vi "Get best pixel array.vi"(9 "Cell details cluster":T1={"Measure?"=TRUE, "Area (cm^2)"=0.0, "Cell Label"="", "Cell Description"="", "Cell Position"=0, "Time in rig (s)"=16.0, "Time to next scan (s)"=0.0, "Scan number"=1.0, "When did you stick it in?"=0.0, "Time between scans (s)"=0.0, "Time of the last scan (s)"=0.0, "Scan settings in queue"=0, "Sample Holder"=0.0, "User Name"=""} {"Scan settings in queue" items=["Regular", "Inverted", "MartinaSettings"]; "Time of the last scan (s)" format="%<%H:%M:%S>t"; "When did you stick it in?" format="%<%H:%M:%S>t"; "Time to next scan (s)" format="%<%H:%M:%S>t"; "Time in rig (s)" format="%<%H:%M:%S>t"}, 10 "Number of best pixels":dbl, 11 "File path of master log":path) -> (2 "Pixel Array":dbl[](array[numeric]), 3 "Vmp Array":dbl[](array[numeric]))   [LabVIEW 2011]
uses:
  Typedefs/Queue cluster.ctl
  <vilib>/Utility/file.llb/Read From Spreadsheet File (string).vi
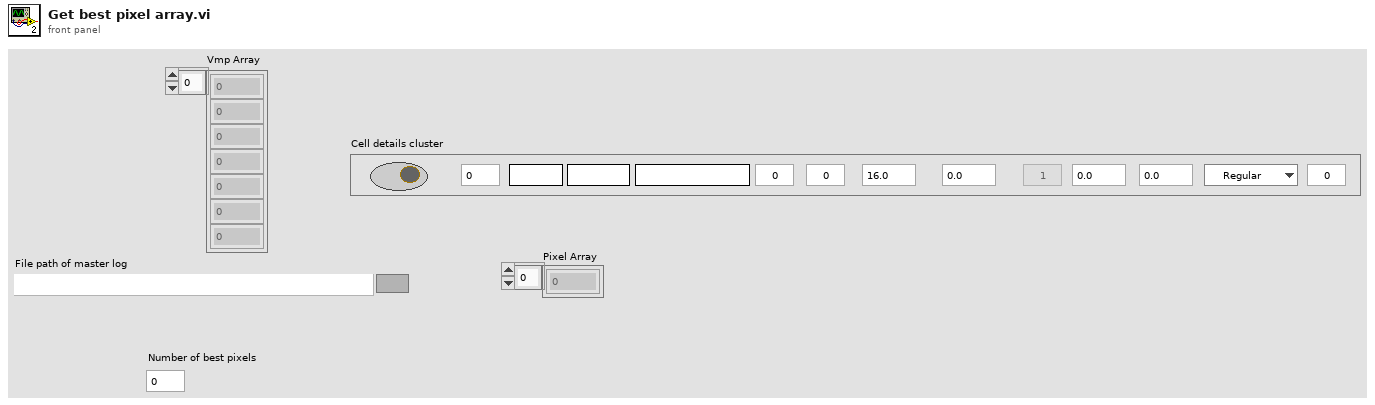
[diagram p1: front panel]
types:
  T1 = typedef "Queue cluster.ctl" = cluster{"Measure?":bool, "Area (cm^2)":dbl, "Cell Label":string, "Cell Description":string, "Cell Position":i32, "Time in rig (s)":dbl, "Time to next scan (s)":dbl, "Scan number":dbl, "When did you stick it in?":dbl, "Time between scans (s)":dbl, "Time of the last scan (s)":dbl, "Scan settings in queue":u16, "Sample Holder":dbl, "User Name":string}
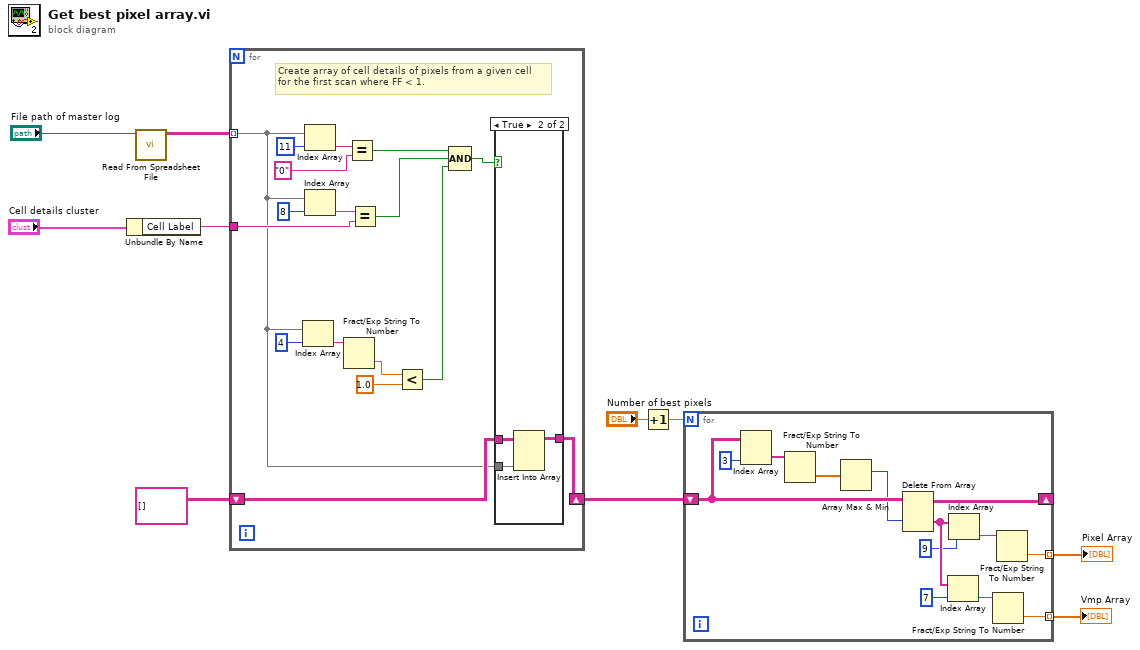
[diagram p0: block diagram]
diagram:
  n1 = Unbundle By Name("Cell details cluster") -> ("Cell Label"=w2:string)
  n2 = call-poly <vilib>:"Read From Spreadsheet File.vi"("file path (dialog if empty)"="File path of master log") -> ("all rows"=w9:string[][])  [unwired: 6 in, 4 out]
  n3 = for {
    tunnel: w9 -> [w12] mode=indexing
    shift-right: [w24] -> w7
    shift-left: string[][] [] ("all rows") -> [w25]
    tunnel: w2 -> [w20]
    # "Create array of cell details of pixels from a given cell\nfor the first scan where FF < 1."
    n4 = Index Array(array=w12, index=4) -> (element=w15:string)
    n5 = Index Array(array=w12, index=11) -> (element=w26:string)
    n6 = Index Array(array=w12, index=8) -> (element=w21:string)
    n7 = Fract/Exp String To Number(string=w15) -> (number=w14:dbl)  [unwired: 3 in, 1 out]
    n8 = Equal?(x=w26, y="0") -> (x = y?=w18:bool)
    n9 = Equal?(x=w21, y=w20) -> (x = y?=w17:bool)
    n10 = Less?(x=w14, y=1.0) -> (x < y?=w11:bool)
    n11 = Compound Arithmetic op=AND(w18, w17, w11) -> (w19:bool)
    n12 = case shown="True" w19 {
      tunnel: w25 -> [w28 w31]
      tunnel: [w28 w30] -> w24
      tunnel: w12 -> [_ w29]
      frame False {
      }
      frame True {
        n13 = Insert Into Array(array=w31, new element=w29) -> (w30:string[][])  [unwired: 2 in]
      }
    }
  }
  n14 = Increment(x="Number of best pixels") -> (x+1=w5:dbl)
  n15 = for {
    N: w5 -> [_]
    shift-right: [w40] -> _
    shift-left: w7 -> [w43]
    tunnel: [w36] -> w4 mode=indexing
    tunnel: [w32] -> w1 mode=indexing
    n16 = Index Array(array=w43, index (col)=3 ("disabled index (col)")) -> (element=w39:string[])  [unwired: 1 in]
    n17 = Fract/Exp String To Number(string=w39) -> (number=w38:dbl[])  [unwired: 3 in, 1 out]
    n18 = Array Max & Min(array=w38) -> (max index (indices)=w42:i32)  [unwired: 3 out]
    n19 = Delete From Array(array=w43, index (row)=w42) -> (deleted portion=w35:string[], array with subset deleted=w40:string[][])  [unwired: 2 in]
    n20 = Index Array(array=w35, index=7) -> (element=w37:string)
    n21 = Index Array(array=w35, index=9) -> (element=w33:string)
    n22 = Fract/Exp String To Number(string=w37) -> (number=w36:dbl)  [unwired: 3 in, 1 out]
    n23 = Fract/Exp String To Number(string=w33) -> (number=w32:dbl)  [unwired: 3 in, 1 out]
  }
  "Vmp Array" <- w4
  "Pixel Array" <- w1
